vi "CRYGet Tree Unicode.vi"() -> (1 "Unicode Message Sub":string[](array[string]))   [LabVIEW 2013]
uses:
  CRYMainGlobal.vi
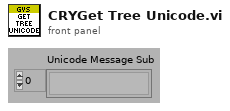
[diagram p1: front panel]
types:
  T1 = enum32{"English", "Chinese", "Korean", "Japanese", "Russian", "Chinese traditional"}
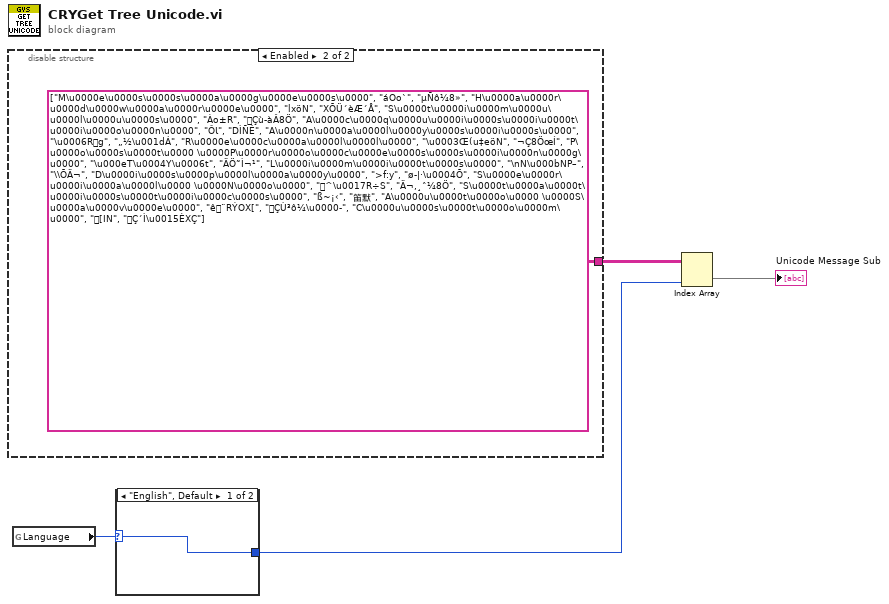
[diagram p0: block diagram]
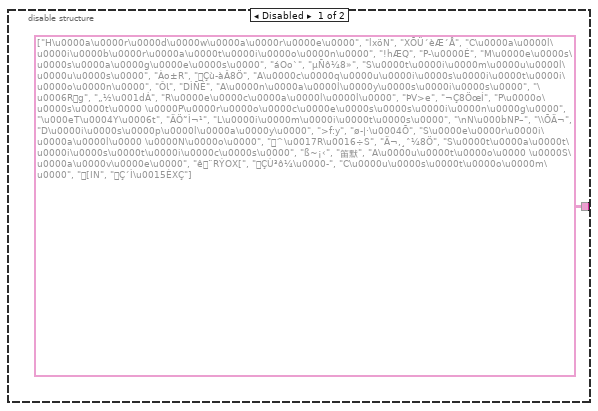
[diagram p2: hidden frame]
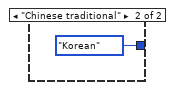
[diagram p3: hidden frame]
diagram:
  n1 = disable-structure shown="Enabled" {
    disable-tunnel: [string[][] [["H\u0000a\u0000r\u0000d\u0000w\u0000a\u0000r\u0000e\u0000", "lxöN", "XÕÜ´èÆ´Å"], ["C\u0000a\u0000l\u0000i\u0000b\u0000r\u0000a\u0000t\u0000i\u0000o\u0000n\u0000", "!hÆQ", "P­\u0000É"], ["M\u0000e\u0000s\u0000s\u0000a\u0000g\u0000e\u0000s\u0000", "áOo`", "µÑô¼8»"], ["S\u0000t\u0000i\u0000m\u0000u\u0000l\u0000u\u0000s\u0000", "Ào±R", "Çù­àÂ8Ö"], ["A\u0000c\u0000q\u0000u\u0000i\u0000s\u0000i\u0000t\u0000i\u0000o\u0000n\u0000", "ǑƖ", "DÌÑÉ"], ["A\u0000n\u0000a\u0000l\u0000y\u0000s\u0000i\u0000s\u0000", "\u0006Rg", "„½\u001dÁ"], ["R\u0000e\u0000c\u0000a\u0000l\u0000l\u0000", "ÞV>e", "¬Ç8ÖœÍ"], ["P\u0000o\u0000s\u0000t\u0000 \u0000P\u0000r\u0000o\u0000c\u0000e\u0000s\u0000s\u0000i\u0000n\u0000g\u0000", "\u000eT\u0004Y\u0006t", "ÄÖ˜Ì¬¹"], ["L\u0000i\u0000m\u0000i\u0000t\u0000s\u0000", "\nN\u000bNP–", "\\ÕÄ¬"], ["D\u0000i\u0000s\u0000p\u0000l\u0000a\u0000y\u0000", ">f:y", "ø­|·\u0004Õ"], ["S\u0000e\u0000r\u0000i\u0000a\u0000l\u0000 \u0000N\u0000o\u0000", "^\u0017R\u0016÷S", "Ä¬,¸ˆ¼8Ö"], ["S\u0000t\u0000a\u0000t\u0000i\u0000s\u0000t\u0000i\u0000c\u0000s\u0000", "ß~¡‹", "笛默"], ["A\u0000u\u0000t\u0000o\u0000 \u0000S\u0000a\u0000v\u0000e\u0000", "ê¨RÝOX[", "ÇÙ³ô¼\u0000­"], ["C\u0000u\u0000s\u0000t\u0000o\u0000m\u0000", "ꁚ[IN", "Ç´Ì\u0015ÈXÇ"]] string[][] [["M\u0000e\u0000s\u0000s\u0000a\u0000g\u0000e\u0000s\u0000", "áOo`", "µÑô¼8»"], ["H\u0000a\u0000r\u0000d\u0000w\u0000a\u0000r\u0000e\u0000", "lxöN", "XÕÜ´èÆ´Å"], ["S\u0000t\u0000i\u0000m\u0000u\u0000l\u0000u\u0000s\u0000", "Ào±R", "Çù­àÂ8Ö"], ["A\u0000c\u0000q\u0000u\u0000i\u0000s\u0000i\u0000t\u0000i\u0000o\u0000n\u0000", "ǑƖ", "DÌÑÉ"], ["A\u0000n\u0000a\u0000l\u0000y\u0000s\u0000i\u0000s\u0000", "\u0006Rg", "„½\u001dÁ"], ["R\u0000e\u0000c\u0000a\u0000l\u0000l\u0000", "\u0003Œ(u‡eöN", "¬Ç8ÖœÍ"], ["P\u0000o\u0000s\u0000t\u0000 \u0000P\u0000r\u0000o\u0000c\u0000e\u0000s\u0000s\u0000i\u0000n\u0000g\u0000", "\u000eT\u0004Y\u0006t", "ÄÖ˜Ì¬¹"], ["L\u0000i\u0000m\u0000i\u0000t\u0000s\u0000", "\nN\u000bNP–", "\\ÕÄ¬"], ["D\u0000i\u0000s\u0000p\u0000l\u0000a\u0000y\u0000", ">f:y", "ø­|·\u0004Õ"], ["S\u0000e\u0000r\u0000i\u0000a\u0000l\u0000 \u0000N\u0000o\u0000", "^\u0017R÷S", "Ä¬,¸ˆ¼8Ö"], ["S\u0000t\u0000a\u0000t\u0000i\u0000s\u0000t\u0000i\u0000c\u0000s\u0000", "ß~¡‹", "笛默"], ["A\u0000u\u0000t\u0000o\u0000 \u0000S\u0000a\u0000v\u0000e\u0000", "ê¨RÝOX[", "ÇÙ³ô¼\u0000­"], ["C\u0000u\u0000s\u0000t\u0000o\u0000m\u0000", "ꁚ[IN", "Ç´Ì\u0015ÈXÇ"]]] -> w4
    frame Disabled {
    }
    frame Enabled {
    }
  }
  n2 = global read "CRYMainGlobal.vi" "Language"() -> (w1:T1)
  n3 = case shown="\"English\", Default" w1 {
    selector: w1 -> [w7 _]
    tunnel: [w7 T1."Korean" ("Language")] -> w3
    frame "English", Default {
    }
    frame "Chinese traditional" {
    }
  }
  n4 = Index Array(array=w4, index (col)=w3) -> (element=→"Unicode Message Sub":string[])  [unwired: 1 in]
